vi "Day 3.1 - .vi"(11 "input":string[](array[string])) -> (3 "output":i16)   [LabVIEW 2021]
uses:
  e8bff944-bf3f-47bc-8a5c-25c6f3011f65.vi
  f6b0d727-c6a6-40eb-9f8f-d9afa3b08fc4.vi
  <vilib>/Comparison/Less/Less Functor/Less Functor.lvclass
  <vilib>/regexp/Match Regular Expression.xnode
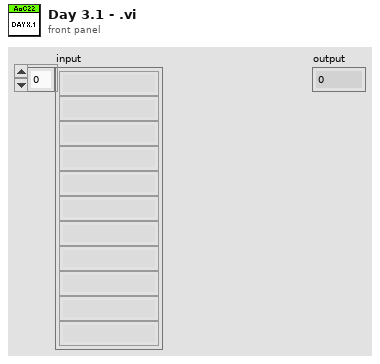
[diagram p1: front panel]
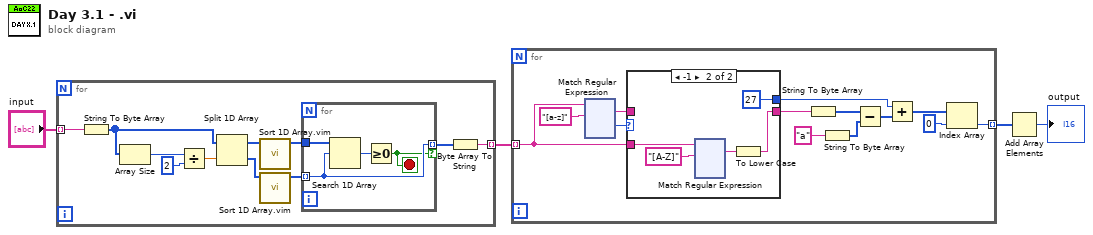
[diagram p0: block diagram]
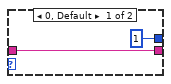
[diagram p2: hidden frame]
diagram:
  n1 = for {
    tunnel: "input" -> [w9] mode=indexing
    tunnel: [w6] -> w3 mode=indexing
    n2 = String To Byte Array(string=w9) -> (unsigned byte array=w14:u8[])
    n3 = Array Size(array=w14) -> (size(s)=w15:i32)
    n4 = Divide(x=w15, y=2) -> (x/y=w13:dbl)
    n5 = Split 1D Array(array=w14, index=w13) -> (first subarray=w11:u8[], second subarray=w10:u8[])
    n6 = call "Sort 1D Array.vim"("unsorted array"=w11) -> ("sorted array"=w7:u8[])  [unwired: 10 in]
    n7 = call "Sort 1D Array.vim"("unsorted array"=w10) -> ("sorted array"=w8:u8[])  [unwired: 10 in]
    n8 = for {
      tunnel: w8 -> [w17] mode=indexing
      tunnel: w7 -> [w19]
      tunnel: [w17] -> w5 mode=indexing if=w16
      stop <- w16 stop-if-true
      n9 = Search 1D Array(1D array=w19, element=w17) -> (index of element=w18:i32)  [unwired: 1 in]
      n10 = Greater Or Equal To 0?(x=w18) -> (x >= 0?=w16:bool)
    }
    n11 = Byte Array To String(unsigned byte array=w5) -> (string=w6:string)
  }
  n12 = for {
    tunnel: w3 -> [w30] mode=indexing
    tunnel: [w22] -> w2 mode=indexing
    n13 = xnode "Match Regular Expression"("input string"=w30, "regular expression"="[a-z]") -> ("whole match"=w20:string, "offset past match"=w31:i32)  [unwired: 4 in, 3 out]
    n14 = case shown="-1" w31 {
      tunnel: w30 -> [_ w38]
      tunnel: [1 27] -> w25
      tunnel: [w34 w36] -> w26
      tunnel: w20 -> [w34 _]
      frame 0, Default {
      }
      frame -1 {
        n15 = xnode "Match Regular Expression"("input string"=w38, "regular expression"="[A-Z]") -> ("whole match"=w35:string)  [unwired: 4 in, 4 out]
        n16 = To Lower Case(string=w35) -> (all lower case string=w36:string)
      }
    }
    n17 = String To Byte Array(string=w26) -> (unsigned byte array=w29:u8[])
    n18 = String To Byte Array(string="a" ("regular expression")) -> (unsigned byte array=w27:u8[])
    n19 = Subtract(x=w29, y=w27) -> (x-y=w24:u8[])
    n20 = Add(x=w25, y=w24) -> (x+y=w23:i32[])
    n21 = Index Array(array=w23, index=0) -> (element=w22:i32)
  }
  n22 = Add Array Elements(numeric array=w2) -> (sum=→"output":i32)
